vi "Actor Core.vi"(8 "error in":errorcluster, 11 "Controller in":refnum<class "Controller.lvclass">) -> (0 "error out":errorcluster, 3 "Actor out":refnum<class "Actor.lvclass">)   [LabVIEW 2013, in "Controller.lvlib" / "Controller.lvclass"]
doc: "(<B>Filename</B>: Actor Framework.lvlib:Actor.lvclass:Actor Core.vi)\n\nReceives messages to the actor, reacts to them, and initiates any error handling that may shut the actor down.\n\nDescendant classes may override this VI to append parallel tasks for the actor to complete while it handles messages. Overrides use the Call Parent Method node."
uses:
  Controller.lvclass
  <vilib>/ActorFramework/Actor/Actor.lvclass
  Operators/Addition/Addition.lvclass
  Operators/Divide/Divide.lvclass
  Operators/Multiply/Multiply.lvclass
  Operators/Subtraction/Subtraction.lvclass
  <vilib>/ActorFramework/Message Queue/Message Queue.lvclass/Message Queue.ctl
  Controller.lvclass/Controller.ctl
  <vilib>/ActorFramework/Stop Msg/Stop Msg.lvclass/Stop Msg.ctl
  <vilib>/ActorFramework/Message Enqueuer/Message Enqueuer.lvclass/Message Enqueuer.ctl
  <vilib>/ActorFramework/Message Enqueuer/Enqueue Critical.vi
  <vilib>/ActorFramework/Message Priority Queue/Priority Enqueue.vi
  <vilib>/ActorFramework/Message Enqueuer/Message Enqueuer.lvclass
  <vilib>/ActorFramework/Stop Msg/Stop Msg.lvclass
  <vilib>/ActorFramework/Message Queue/Message Queue.lvclass
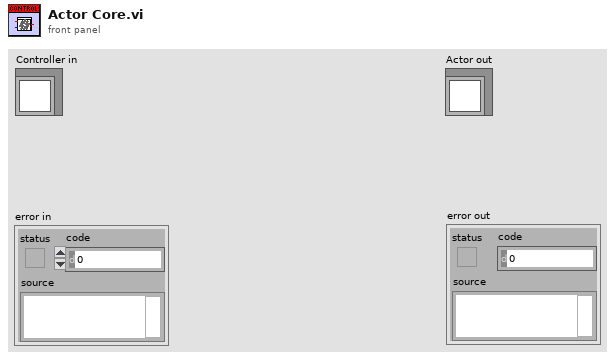
[diagram p1: front panel]
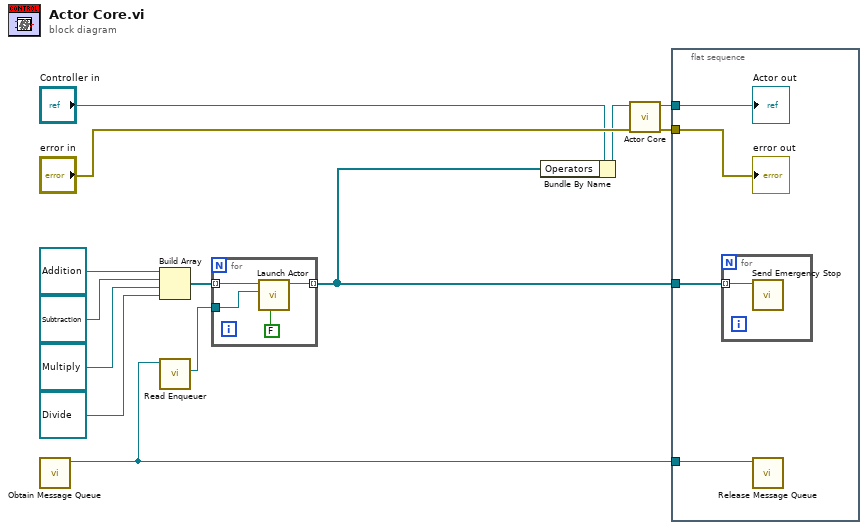
[diagram p0: block diagram]
diagram:
  n1 = call <vilib>:"Obtain Message Queue.vi"() -> ("Message Queue"=w9:refnum<class "Message Queue.lvclass">)  [unwired: 10 in, 1 out]
  n2 = Build Array(refnum<class "Addition.lvclass"> refnum ("Operators.lvlib:Addition.lvclass"), refnum<class "Subtraction.lvclass"> refnum ("Operators.lvlib:Subtraction.lvclass"), refnum<class "Multiply.lvclass"> refnum ("Operators.lvlib:Multiply.lvclass"), refnum<class "Divide.lvclass"> refnum ("Operators.lvlib:Divide.lvclass")) -> (w5:refnum<class "Calculate.lvclass">[])
  n3 = call <vilib>:"Read Enqueuer.vi"("Message Queue"=w9) -> ("Message Enqueuer"=w6:refnum<class "Message Enqueuer.lvclass">)  [unwired: 10 in]
  n4 = for {
    tunnel: w5 -> [w17] mode=indexing
    tunnel: w6 -> [w16]
    tunnel: [w15] -> w7 mode=indexing
    n5 = call <vilib>:"Launch Actor.vi"("Open Actor Core front panel? (F)"=FALSE, "Actor-to-Caller Enqueuer"=w16, "Actor"=w17) -> ("Caller-To-Actor Enqueuer"=w15:refnum<class "Message Enqueuer.lvclass">)  [unwired: 7 in, 1 out]
  }
  n6 = Bundle By Name(cluster="Controller in", "Operators"=w7) -> (w8:refnum<class "Controller.lvclass">)
  n7 = call-parent "Actor Core.vi"("error in"="error in", "Actor in"=w8) -> ("error out"=w13:errorcluster, "Actor out"=w12:refnum<class "Actor.lvclass">)  [unwired: 8 in]
  n8 = flat-sequence {
    tunnel: w13 -> [w21]
    tunnel: w12 -> [w20]
    tunnel: w7 -> [w18]
    tunnel: w9 -> [w19]
    frame #0 {
      n9 = for {
        tunnel: w18 -> [w22] mode=indexing
        n10 = call <vilib>:"Send Emergency Stop.vi"("Message Enqueuer"=w22) -> ()  [unwired: 10 in, 1 out]
      }
      n11 = call <vilib>:"Release Message Queue.vi"("Message Queue"=w19) -> ()  [unwired: 9 in, 2 out]
      "error out" <- w21
      "Actor out" <- w20
    }
  }
